vi "digitally_ros_without_joystick_init_val_WORKING.vi"() -> ()   [LabVIEW 2019]
uses:
  <vilib>/addons/eal4LabVIEW/ApiLib/Connection control/ealApiConnect_string.vi
  <vilib>/addons/eal4LabVIEW/eal4LabVIEW.lvlib
panel:
  out "Iteration counter loop 1":i32
  out "Init success\\fail":i32
  out "Diviation 3":dbl
  out "Diviation 2":dbl
  out "Diviation 1":dbl
  out "Sensor values":dbl[](array[numeric])
  out "List length":i32
  in  "stop 3":bool
  in  "stop 2":bool
  out "I value (loop 3)":i32
  out "Is the PID fnished?":bool[](array[boolean])
  out "In Range? (1)":bool
  out "In Range? (2)":bool
  out "In Range? (3)":bool
  in  "condition 6":i32(ring) items=["AXIS_CONDITION_ACTIVE"=0, "AXIS_CONDITION_PARKING"=1, "AXIS_CONDITION_DEACTIVATED"=2, "AXIS_CONDITION_ACTIVE_DECOUPLED"=4, "AXIS_CONDITION_PARKING_DECOUPLED"=5, "AXIS_CONDITION_DEACTIVATED_DECOUPLED"=6, "AXIS_CONDITION_ACTIVE_PARAMETERIZATION"=8, "AXIS_CONDITION_PARKING_PARAMETERIZATION"=9, "AXIS_CONDITION_DEACTIVATED_PARAMETERIZATION"=10, "AXIS_CONDITION_ACTIVE_DECOUPLED_PARAMETERIZATION"=12, "AXIS_CONDITION_PARKING_DECOUPLED_PARAMETERIZATION"=13, "AXIS_CONDITION_DEACTIVATED_DECOUPLED_PARAMETERIZATION"=14]
  in  "slave index 6":i32
  in  "condition 5":i32(ring) items=["AXIS_CONDITION_ACTIVE"=0, "AXIS_CONDITION_PARKING"=1, "AXIS_CONDITION_DEACTIVATED"=2, "AXIS_CONDITION_ACTIVE_DECOUPLED"=4, "AXIS_CONDITION_PARKING_DECOUPLED"=5, "AXIS_CONDITION_DEACTIVATED_DECOUPLED"=6, "AXIS_CONDITION_ACTIVE_PARAMETERIZATION"=8, "AXIS_CONDITION_PARKING_PARAMETERIZATION"=9, "AXIS_CONDITION_DEACTIVATED_PARAMETERIZATION"=10, "AXIS_CONDITION_ACTIVE_DECOUPLED_PARAMETERIZATION"=12, "AXIS_CONDITION_PARKING_DECOUPLED_PARAMETERIZATION"=13, "AXIS_CONDITION_DEACTIVATED_DECOUPLED_PARAMETERIZATION"=14]
  in  "slave index 5":i32
  in  "condition 4":i32(ring) items=["AXIS_CONDITION_ACTIVE"=0, "AXIS_CONDITION_PARKING"=1, "AXIS_CONDITION_DEACTIVATED"=2, "AXIS_CONDITION_ACTIVE_DECOUPLED"=4, "AXIS_CONDITION_PARKING_DECOUPLED"=5, "AXIS_CONDITION_DEACTIVATED_DECOUPLED"=6, "AXIS_CONDITION_ACTIVE_PARAMETERIZATION"=8, "AXIS_CONDITION_PARKING_PARAMETERIZATION"=9, "AXIS_CONDITION_DEACTIVATED_PARAMETERIZATION"=10, "AXIS_CONDITION_ACTIVE_DECOUPLED_PARAMETERIZATION"=12, "AXIS_CONDITION_PARKING_DECOUPLED_PARAMETERIZATION"=13, "AXIS_CONDITION_DEACTIVATED_DECOUPLED_PARAMETERIZATION"=14]
  in  "slave index 4":i32
  out "RPM 1 ROS":dbl
  out "RPM 2 ROS":dbl
  out "RPM 3 ROS":dbl
  in  "stop 1":bool
  out "Return value":dbl[](array[numeric])
  out "Iteration counter loop 2":i32
  # "ROS Control"
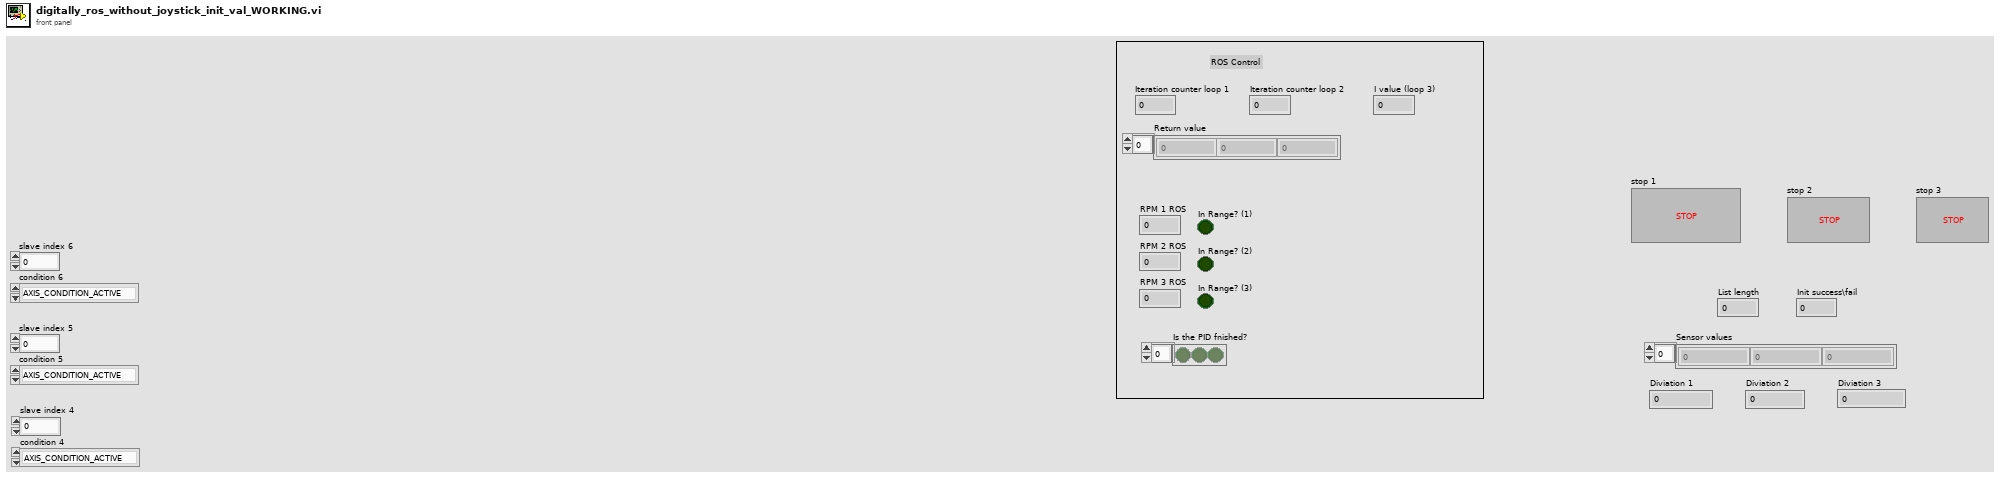
[diagram p1: front panel]
types:
  T1 = cluster{"Velocity":dbl, "Acceleration":dbl, "Deceleration":dbl, "Jerk":dbl}
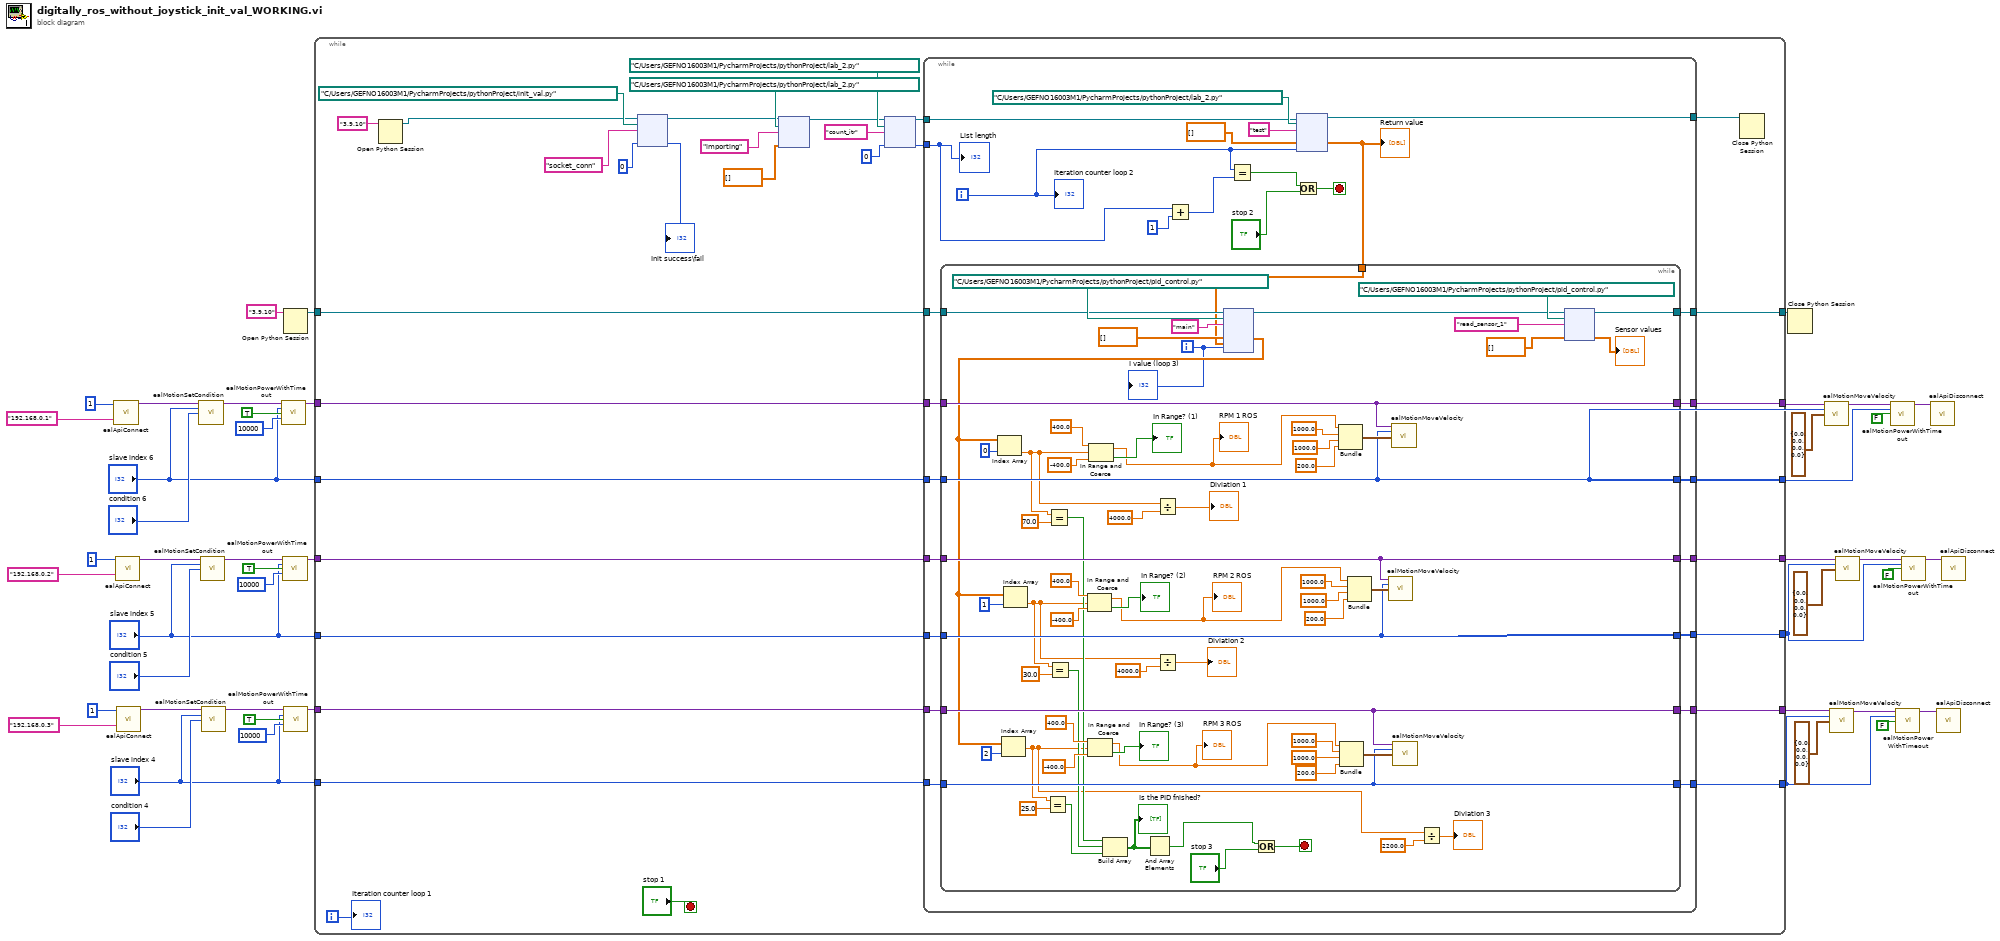
[diagram p0: block diagram]
diagram:
  n1 = call-poly <vilib>:"ealApiConnect.vi"("maximum no of axes"=1, "ip address"="192.168.0.1") -> ("connection out"=w20:variant)  [unwired: 12 in, 1 out]
  n2 = call-poly <vilib>:"ealApiConnect.vi"("maximum no of axes"=1, "ip address"="192.168.0.2") -> ("connection out"=w27:variant)  [unwired: 12 in, 1 out]
  n3 = call-poly <vilib>:"ealApiConnect.vi"("maximum no of axes"=1, "ip address"="192.168.0.3") -> ("connection out"=w34:variant)  [unwired: 12 in, 1 out]
  n4 = call <vilib>:"ealMotionSetCondition.vi"("connection in"=w20, "slave index"="slave index 6", "condition"="condition 6") -> ("connection out"=w19:variant)  [unwired: 11 in, 1 out]
  n5 = call <vilib>:"ealMotionSetCondition.vi"("connection in"=w27, "slave index"="slave index 5", "condition"="condition 5") -> ("connection out"=w26:variant)  [unwired: 11 in, 1 out]
  n6 = call <vilib>:"ealMotionSetCondition.vi"("connection in"=w34, "slave index"="slave index 4", "condition"="condition 4") -> ("connection out"=w33:variant)  [unwired: 11 in, 1 out]
  n7 = call <vilib>:"ealMotionPowerWithTimeout.vi"("connection in"=w19, "slave index"="slave index 6", "value"=TRUE, "timeout"=10000) -> ("connection out"=w15:variant)  [unwired: 10 in, 1 out]
  n8 = call <vilib>:"ealMotionPowerWithTimeout.vi"("connection in"=w26, "slave index"="slave index 5", "value"=TRUE, "timeout"=10000) -> ("connection out"=w14:variant)  [unwired: 10 in, 1 out]
  n9 = Open Python Session(python version="3.9.10" ("Python version")) -> (session out=w4:refnum<k35>)  [unwired: 2 in, 1 out]
  n10 = call <vilib>:"ealMotionPowerWithTimeout.vi"("connection in"=w33, "slave index"="slave index 4", "value"=TRUE, "timeout"=10000) -> ("connection out"=w13:variant)  [unwired: 10 in, 1 out]
  n11 = while {
    tunnel: w15 -> [w80]
    tunnel: w14 -> [w79]
    tunnel: w13 -> [w78]
    tunnel: [w67] -> w12
    tunnel: [w77] -> w11
    tunnel: "slave index 6" -> [w76]
    tunnel: "slave index 5" -> [w75]
    tunnel: [w74] -> w8
    tunnel: [w70] -> w7
    tunnel: "slave index 4" -> [w73]
    tunnel: w4 -> [w72]
    tunnel: [w68] -> w3
    tunnel: [w71] -> w2
    tunnel: [w69] -> w1
    i -> [w52]
    stop <- "stop 1" stop-if-true
    n12 = Open Python Session(python version="3.9.10" ("Python version")) -> (session out=w50:refnum<k35>)  [unwired: 2 in, 1 out]
    n13 = node(w50, path "C:/Users/GEFNO16003M1/PycharmProjects/pythonProject/init_val.py" ("module path"), "socket_conn" ("function name"), 0) -> (w55:refnum<k35>, →"Init success\\fail":i32)  [unwired: 1 in, 3 out]
    n14 = node(w55, path "C:/Users/GEFNO16003M1/PycharmProjects/pythonProject/lab_2.py" ("module path"), "importing" ("function name"), dbl[] []) -> (w61:refnum<k35>)  [unwired: 2 in, 3 out]
    n15 = node(w61, path "C:/Users/GEFNO16003M1/PycharmProjects/pythonProject/lab_2.py" ("module path"), "count_itr" ("function name"), 0) -> (w60:refnum<k35>, w58:i32)  [unwired: 1 in, 3 out]
    n16 = while {
      tunnel: [w104] -> w49
      tunnel: w60 -> [w106]
      tunnel: w58 -> [w83]
      tunnel: w80 -> [w102]
      tunnel: w79 -> [w92]
      tunnel: w78 -> [w101]
      tunnel: [w94] -> w67
      tunnel: [w95] -> w77
      tunnel: w76 -> [w93]
      tunnel: w75 -> [w91]
      tunnel: [w96] -> w74
      tunnel: w73 -> [w98]
      tunnel: w72 -> [w90]
      tunnel: [w100] -> w68
      tunnel: [w99] -> w71
      tunnel: [w97] -> w70
      tunnel: [w89] -> w69
      i -> [w82]
      stop <- w88 stop-if-true
      n17 = Add(x=w83, y=1) -> (x+y=w85:i32)
      n18 = Equal?(x=w82, y=w85) -> (x = y?=w86:bool)
      n19 = Or(x=w86, y="stop 2") -> (x .or. y?=w88:bool)
      n20 = node(w106, path "C:/Users/GEFNO16003M1/PycharmProjects/pythonProject/lab_2.py" ("module path"), "test" ("function name"), dbl[] [], w82) -> (w104:refnum<k35>, w103:dbl[])  [unwired: 2 in, 3 out]
      "Return value" <- w103
      n21 = while {
        tunnel: w103 -> [w124]
        tunnel: w102 -> [w144]
        tunnel: w101 -> [w146]
        tunnel: [w146] -> w100
        tunnel: [w145] -> w99
        tunnel: w98 -> [w145]
        tunnel: [w142] -> w97
        tunnel: [w141] -> w96
        tunnel: [w143] -> w95
        tunnel: [w144] -> w94
        tunnel: w93 -> [w143]
        tunnel: w92 -> [w142]
        tunnel: w91 -> [w141]
        tunnel: w90 -> [w140]
        tunnel: [w123] -> w89
        i -> [w128]
        stop <- w127 stop-if-true
        n22 = node(w140, path "C:/Users/GEFNO16003M1/PycharmProjects/pythonProject/pid_control.py" ("module path"), "main" ("function name"), dbl[] [], w124, w128) -> (w118:refnum<k35>, w139:dbl[])  [unwired: 3 in, 3 out]
        n23 = Index Array(array=w139, index=0) -> (element=w117:dbl)
        n24 = Index Array(array=w139, index=2) -> (element=w111:dbl)
        n25 = Index Array(array=w139, index=1) -> (element=w114:dbl)
        n26 = Equal?(x=w111, y=25.0) -> (x = y?=w133:bool)
        n27 = Equal?(x=w117, y=70.0) -> (x = y?=w135:bool)
        n28 = Equal?(x=w114, y=30.0) -> (x = y?=w134:bool)
        n29 = In Range and Coerce(upper limit=400.0, x=w114, lower limit=-400.0) -> (coerced(x)=w130:dbl, In Range?=→"In Range? (2)":bool)
        "RPM 2 ROS" <- w130
        n30 = In Range and Coerce(upper limit=400.0, x=w111, lower limit=-400.0) -> (coerced(x)=w129:dbl, In Range?=→"In Range? (3)":bool)
        "RPM 3 ROS" <- w129
        n31 = In Range and Coerce(upper limit=400.0, x=w117, lower limit=-400.0) -> (coerced(x)=w131:dbl, In Range?=→"In Range? (1)":bool)
        "RPM 1 ROS" <- w131
        n32 = Build Array(w135, w134, w133) -> (w132:bool[])
        "Is the PID fnished?" <- w132
        n33 = And Array Elements(Boolean array=w132) -> (logical AND=w126:bool)
        n34 = Divide(x=w117, y=4000.0) -> (x/y=→"Diviation 1":dbl)
        n35 = Divide(x=w114, y=4000.0) -> (x/y=→"Diviation 2":dbl)
        n36 = Or(x=w126, y="stop 3") -> (x .or. y?=w127:bool)
        n37 = Bundle("upper limit"=w131, 1000.0, 1000.0, 200.0) -> (w156:cluster{"upper limit":dbl, dbl, dbl, dbl})  [unwired: 1 in]
        n38 = Bundle("upper limit"=w129, 1000.0, 1000.0, 200.0) -> (w166:cluster{"upper limit":dbl, dbl, dbl, dbl})  [unwired: 1 in]
        n39 = Bundle("upper limit"=w130, 1000.0, 1000.0, 200.0) -> (w161:cluster{"upper limit":dbl, dbl, dbl, dbl})  [unwired: 1 in]
        n40 = call <vilib>:"ealMotionMoveVelocity.vi"("connection in"=w142, "slave index"=w141, "parameters set"=w161) -> ()  [unwired: 11 in, 2 out]
        n41 = call <vilib>:"ealMotionMoveVelocity.vi"("connection in"=w144, "slave index"=w143, "parameters set"=w156) -> ()  [unwired: 11 in, 2 out]
        n42 = call <vilib>:"ealMotionMoveVelocity.vi"("connection in"=w146, "slave index"=w145, "parameters set"=w166) -> ()  [unwired: 11 in, 2 out]
        n43 = Divide(x=w111, y=2200.0) -> (x/y=→"Diviation 3":dbl)
        n44 = node(w118, path "C:/Users/GEFNO16003M1/PycharmProjects/pythonProject/pid_control.py" ("module path"), "read_sensor_1" ("function name"), dbl[] []) -> (w123:refnum<k35>, →"Sensor values":dbl[])  [unwired: 1 in, 3 out]
        "I value (loop 3)" <- w128
      }
      "Iteration counter loop 2" <- w82
      "List length" <- w83
    }
    n45 = Close Python Session(session in=w49) -> ()  [unwired: 1 in, 1 out]
    "Iteration counter loop 1" <- w52
  }
  n46 = Close Python Session(session in=w1) -> ()  [unwired: 1 in, 1 out]
  n47 = call <vilib>:"ealMotionMoveVelocity.vi"("connection in"=w12, "slave index"=w11, "parameters set"=T1 {"Velocity"=0.0, "Acceleration"=0.0, "Deceleration"=0.0, "Jerk"=0.0}) -> ("connection out"=w39:variant)  [unwired: 11 in, 1 out]
  n48 = call <vilib>:"ealMotionMoveVelocity.vi"("connection in"=w3, "slave index"=w2, "parameters set"=T1 {"Velocity"=0.0, "Acceleration"=0.0, "Deceleration"=0.0, "Jerk"=0.0}) -> ("connection out"=w47:variant)  [unwired: 11 in, 1 out]
  n49 = call <vilib>:"ealMotionMoveVelocity.vi"("connection in"=w7, "slave index"=w8, "parameters set"=T1 {"Velocity"=0.0, "Acceleration"=0.0, "Deceleration"=0.0, "Jerk"=0.0}) -> ("connection out"=w43:variant)  [unwired: 11 in, 1 out]
  n50 = call <vilib>:"ealMotionPowerWithTimeout.vi"("connection in"=w39, "slave index"=w11, "value"=FALSE) -> ("connection out"=w40:variant)  [unwired: 11 in, 1 out]
  n51 = call <vilib>:"ealMotionPowerWithTimeout.vi"("connection in"=w47, "slave index"=w2, "value"=FALSE) -> ("connection out"=w48:variant)  [unwired: 11 in, 1 out]
  n52 = call <vilib>:"ealMotionPowerWithTimeout.vi"("connection in"=w43, "slave index"=w8, "value"=FALSE) -> ("connection out"=w44:variant)  [unwired: 11 in, 1 out]
  n53 = call <vilib>:"ealApiDisconnect.vi"("connection in"=w40) -> ()  [unwired: 14 in, 1 out]
  n54 = call <vilib>:"ealApiDisconnect.vi"("connection in"=w48) -> ()  [unwired: 14 in, 1 out]
  n55 = call <vilib>:"ealApiDisconnect.vi"("connection in"=w44) -> ()  [unwired: 14 in, 1 out]
